vi "BIO_write.vi"(8 "error in (no error)":errorcluster, 9 "Timeout (10000ms)":u32=10000, 10 "Bytes to write":u8[](array[numeric]), 11 "BIO in":refnum<class "BIO.lvclass">) -> (0 "error out":errorcluster, 2 "Bytes written":i32, 3 "BIO out":refnum<class "BIO.lvclass">)   [LabVIEW 2013, in "OpenSSL Socket.lvlib" / "BIO.lvclass"]
uses:
  BIO.lvclass
  SSL-Lib/SSL-Lib.lvclass
panel:
  out "return type":i32
  out "Numeric":i32
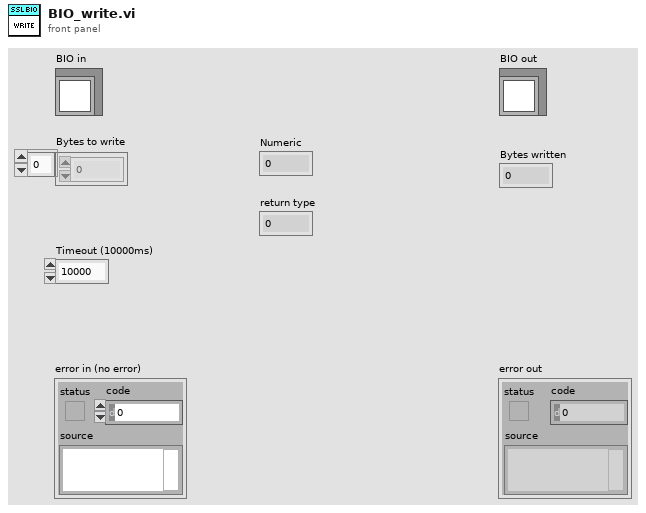
[diagram p1: front panel]
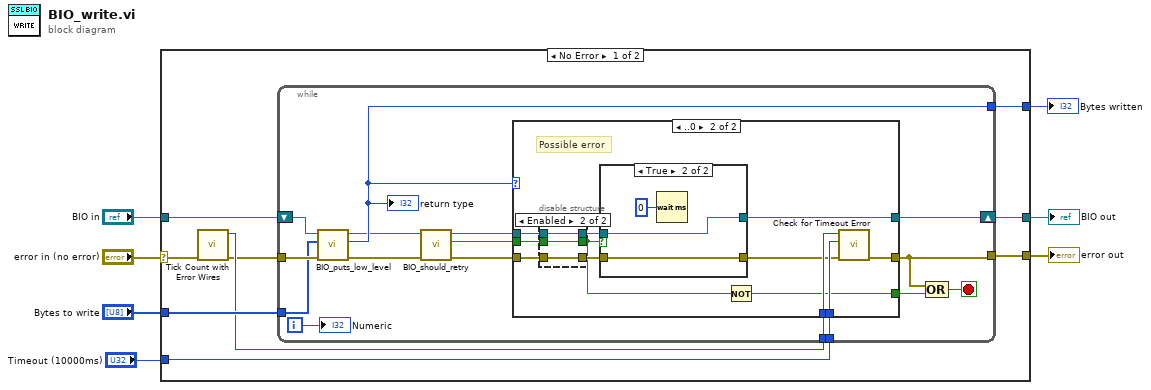
[diagram p0: block diagram]
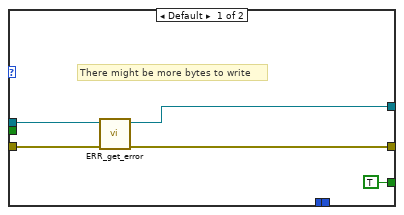
[diagram p2: hidden frame]
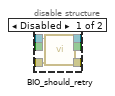
[diagram p3: hidden frame]
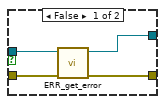
[diagram p4: hidden frame]
diagram:
  n1 = case shown="No Error" "error in (no error)" {
    selector: "error in (no error)" -> [w13 w66]
    tunnel: [w14 w66] -> w6
    tunnel: [w15 w65] -> w4
    tunnel: "BIO in" -> [w9 w65]
    tunnel: "Bytes to write" -> [w16 _]
    tunnel: "Timeout (10000ms)" -> [w11 _]
    tunnel: [w8 _] -> w1
    frame No Error {
      n2 = call "Tick Count with Error Wires.vi"("error in (no error)"=w13) -> ("error out"=w10:errorcluster, "millisecond timer value"=w12:u32)  [unwired: 9 in]
      n3 = while {
        tunnel: w16 -> [w24]
        shift-right: [w31] -> w15
        shift-left: w9 -> [w25]
        tunnel: w10 -> [w32]
        tunnel: [w29] -> w14
        tunnel: w12 -> [w27]
        tunnel: w11 -> [w26]
        tunnel: [w23] -> w8
        i -> [w22]
        stop <- w28 stop-if-true
        n4 = call "BIO_puts_low_level.vi"("error in (no error)"=w32, "Bytes to write"=w24, "BIO in"=w25) -> ("error out"=w21:errorcluster, "return type"=w23:i32, "BIO out"=w19:refnum<class "BIO.lvclass">)  [unwired: 6 in]
        "return type" <- w23
        n5 = call "BIO_should_retry.vi"("error in (no error)"=w21, "BIO in"=w19) -> ("error out"=w20:errorcluster, "Should retry"=w17:bool, "BIO out"=w18:refnum<class "BIO.lvclass">)  [unwired: 7 in]
        n6 = case shown="..0" w23 {
          tunnel: w20 -> [w36 w49]
          tunnel: [w33 w42] -> w29
          tunnel: w18 -> [w35 w48]
          tunnel: [w34 w45] -> w31
          tunnel: [TRUE ("Should retry") w39] -> w30
          tunnel: w27 -> [_ w43]
          tunnel: w26 -> [_ w44]
          tunnel: w17 -> [_ w38]
          frame Default {
            # "There might be more bytes to write"
            n7 = call "ERR_get_error.vi"("error in (no error)"=w36, "SSL-Lib in"=w35) -> ("error out"=w33:errorcluster, "SSL-Lib out"=w34:refnum<class "BIO.lvclass">)  [unwired: 8 in]
          }
          frame ..0 {
            # "Possible error"
            n8 = disable-structure shown="Enabled" {
              disable-tunnel: w49 -> [w54 w57]
              disable-tunnel: w48 -> [w53 w56]
              disable-tunnel: [w52 w57] -> w47
              disable-tunnel: [w51 w56] -> w46
              disable-tunnel: [w50 w55] -> w40
              disable-tunnel: w38 -> [_ w55]
              frame Disabled {
                n9 = call "BIO_should_retry.vi"("error in (no error)"=w54, "BIO in"=w53) -> ("error out"=w52:errorcluster, "Should retry"=w50:bool, "BIO out"=w51:refnum<class "BIO.lvclass">)  [unwired: 7 in]
              }
              frame Enabled {
              }
            }
            n10 = case shown="True" w40 {
              tunnel: w47 -> [w61 w63]
              tunnel: [w60 w63] -> w41
              tunnel: w46 -> [w59 w64]
              tunnel: [w58 w64] -> w45
              frame False {
                n11 = call "ERR_get_error.vi"("error in (no error)"=w61, "SSL-Lib in"=w59) -> ("error out"=w60:errorcluster, "SSL-Lib out"=w58:refnum<class "BIO.lvclass">)  [unwired: 8 in]
              }
              frame True {
                n12 = Wait (ms)(milliseconds to wait=u32 0) -> ()  [unwired: 1 out]
              }
            }
            n13 = Not(x=w40) -> (.not. x?=w39:bool)
            n14 = call "Check for Timeout Error.vi"("error in (no error)"=w41, "Timeout (10000ms)"=w44, "t0"=w43) -> ("error out"=w42:errorcluster)  [unwired: 8 in]
          }
        }
        n15 = Compound Arithmetic op=OR(w29, w30) -> (w28:bool)
        "Numeric" <- w22
      }
    }
    frame Error {
    }
  }
  "error out" <- w6
  "BIO out" <- w4
  "Bytes written" <- w1
